vi "Frame Page.vi"(8 "error in (no error)":errorcluster, 11 "Node Ptr":T2 format="%.0x") -> (0 "error out":errorcluster)   [LabVIEW 2019, in "Protection and Counter Addon System Explorer.lvlib"]
uses:
  Protection and Counter Addon System Explorer.lvlib
  <vilib>/NI VeriStand/Custom Device API/Custom Device Item Ref.ctl
  NationalInstruments.VeriStand.SystemStorageUI
  Types/Event Trigger Type.ctl
  <vilib>/NI VeriStand/UI Controls/Single Node Browser/Net Event Data.ctl
  <vilib>/NI VeriStand/UI Controls/Single Node Browser/Net Event.ctl
  Addon Shared/SubVIs/GUID Lookup.vi
  <vilib>/NI VeriStand/Custom Device API/Custom Device API.lvlib
  <vilib>/NI VeriStand/UI Controls/Single Node Browser/NI_VS UI Single Node Browser.lvlib
  Addon Shared/Protection and Counter Addon Shared.lvlib
panel:
  in  "Transmit Trigger":T1
  in  "Trigger":refnum<k24>(container)
  in  "Trigger Settings":cluster{"Section Name":string}={"Section Name"="Transmission Trigger"}
  in  "Trigger":refnum<k24>(container)
  in  "Disable Transmission":bool
  in  "Disable Settings":cluster{"Section Name":string}={"Section Name"="Disable Transmission"}
  in  "Description":string
  out "Frame ID":u32 format="%.0x"
  in  "Custom Device Settings":cluster{"Section Name":string}={"Section Name"="Custom Device Item Settings"}
  out "Name":string
  in  "SHDocVw.IWebBrowser2":refnum<k7>(container)
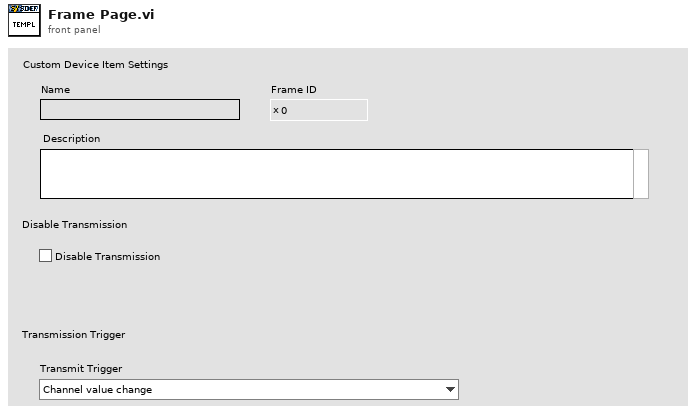
[diagram p1: front panel]
types:
  T1 = typedef "Protection and Counter Addon System Explorer.lvlib/Event Trigger Type.ctl" = enum16{"Channel value change", "Trigger channel (not zero)", "Channel value change or trigger channel (not zero)", "Trigger channel (any value change)", "Channel value change or trigger channel (any value change)"}
  T2 = typedef "Custom Device API.lvlib/Custom Device Item Ref.ctl" = u64
  T3 = cluster{"Trigger":refnum<user-event>, "Transmission":refnum<user-event>}
  T4 = typedef "Protection and Counter Addon System Explorer.lvlib/Frame Settings.ctl" = cluster{"ID":u32, "Disable Transmission":bool, "Disable Transmission Ref":T2, "Transmit Trigger":T1, "Transmit Trigger Ref":T2}
  T5 = typedef "Custom Device API.lvlib/Custom Device Item Info.ctl" = cluster{"Name":string, "Is Channel":bool, "GUID":string, "Is Waveform":bool}
  T6 = typedef "NI_VS UI Single Node Browser.lvlib/Single Node Browser Ref.ctl" = refnum<k24>
  T7 = typedef "NI_VS UI Single Node Browser.lvlib/Callback Type.ctl" = cluster{"Net Callbacks":refnum<k27>[], "Event":refnum<user-event>}
  T8 = typedef "Custom Device API.lvlib/Custom Device Commands.ctl" = enum16{"Default", "Item renamed", "Shutdown", "Dynamic button pressed"}
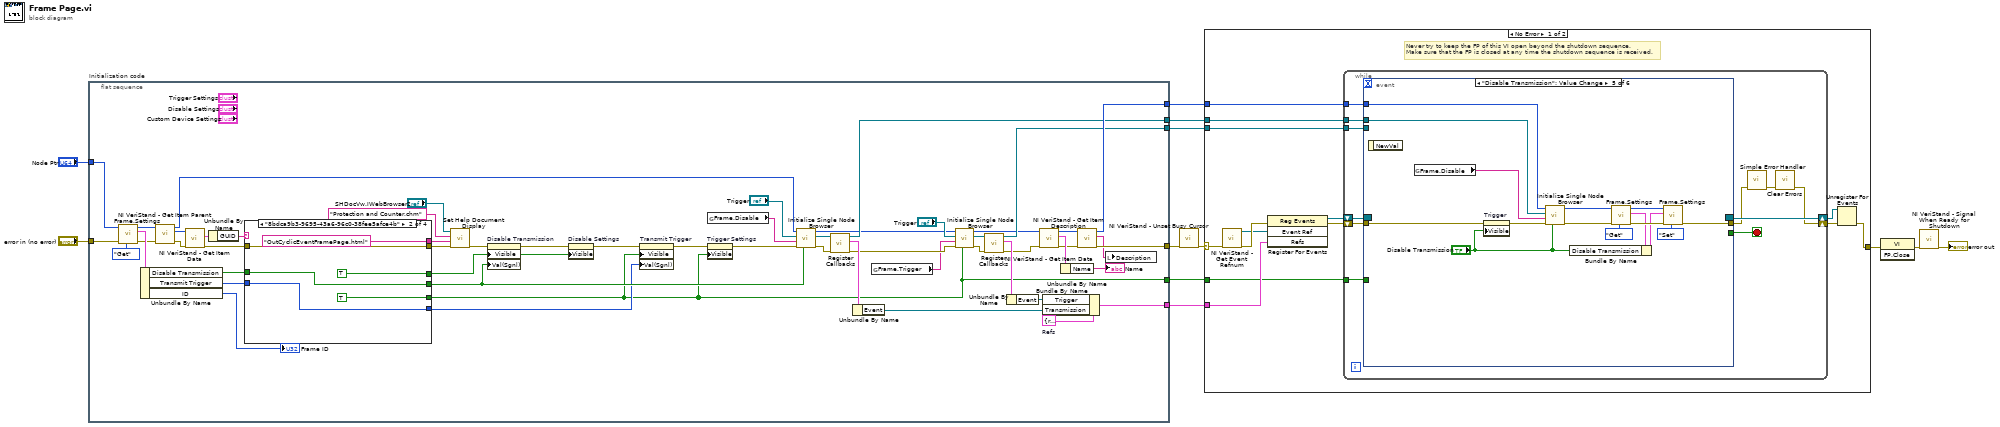
[diagram p0: block diagram]
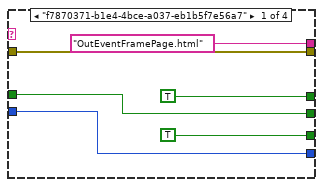
[diagram p2: hidden frame]
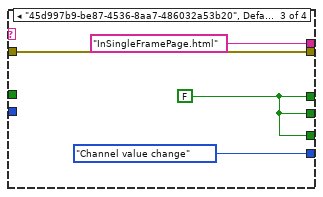
[diagram p3: hidden frame]
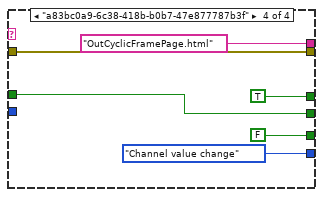
[diagram p4: hidden frame]
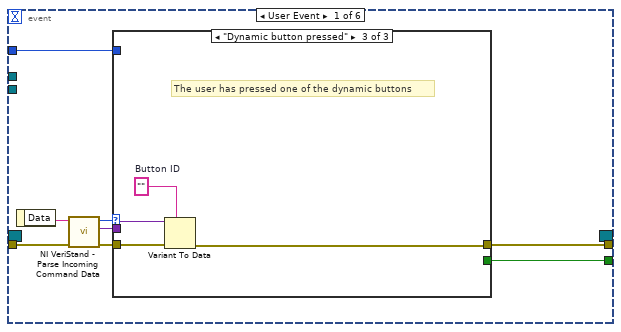
[diagram p5: hidden frame]
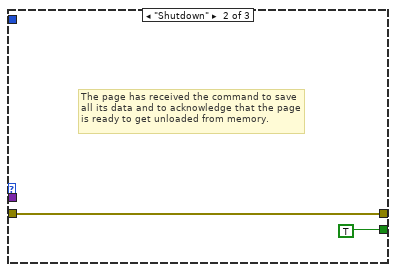
[diagram p7: hidden frame]
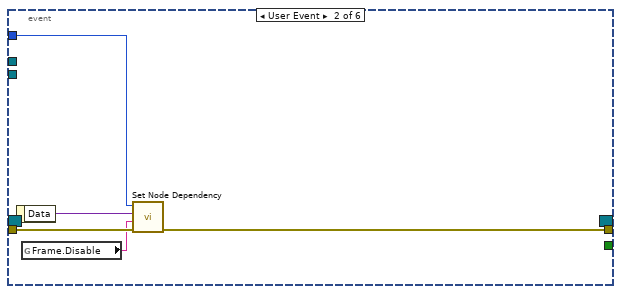
[diagram p8: hidden frame]
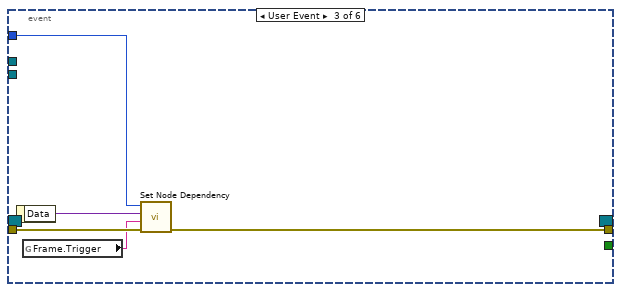
[diagram p9: hidden frame]
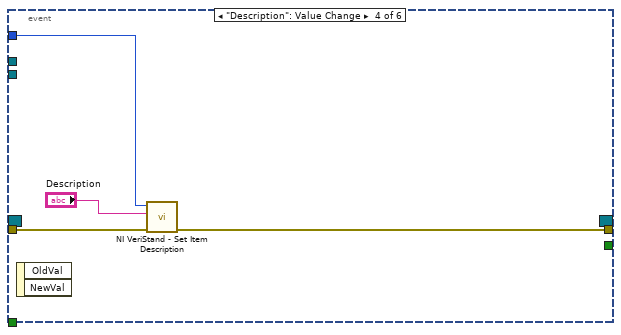
[diagram p10: hidden frame]
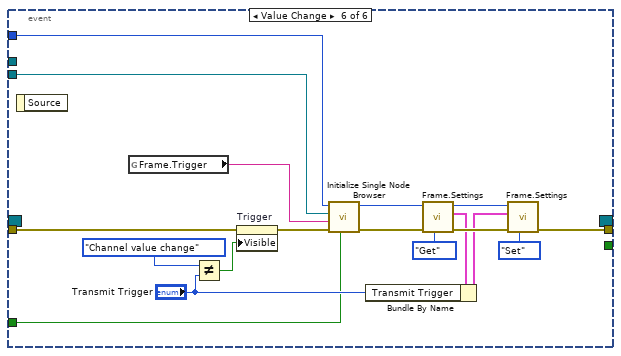
[diagram p11: hidden frame]
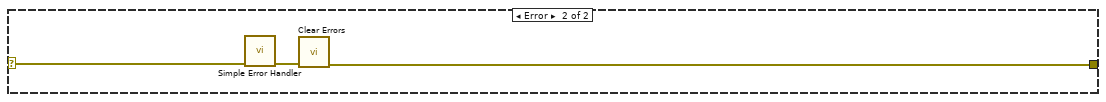
[diagram p12: hidden frame]
diagram:
  n1 = flat-sequence "Initialization code" {
    tunnel: "error in (no error)" -> [w22]
    tunnel: "Node Ptr" -> [w20]
    tunnel: [w61] -> w7
    tunnel: [w59] -> w5
    tunnel: [w43] -> w4
    tunnel: [w45] -> w3
    tunnel: [w35] -> w2
    tunnel: [w15] -> w1
    frame #0 {
      w38 = T3 {"Trigger"=refnum, "Transmission"=refnum}  # Refs
      n2 = call "Frame.Settings.vi"("Action"=enum8{"Get", "Set"}."Get", "error in (no error)"=w22, "Item Ref in"=w20) -> ("error out"=w21:errorcluster, "Frame.Settings"=w26:T4, "Item Ref out"=w19:T2)  [unwired: 6 in]
      n3 = Unbundle By Name(w26) -> ("Disable Transmission"=w18:bool, "Transmit Trigger"=w17:T1, "ID"=→"Frame ID":u32)
      n4 = call <vilib>:"NI VeriStand - Get Item Parent.vi"("error in (no error)"=w21, "Item Ref in"=w19) -> ("error out"=w57:errorcluster, "Parent Ref"=w56:T2, "Item Ref out"=w49:T2)  [unwired: 6 in, 1 out]
      n5 = call <vilib>:"NI VeriStand - Get Item Data.vi"("error in (no error)"=w57, "Item Ref in"=w56) -> ("error out"=w53:errorcluster, "Item Info"=w55:T5)  [unwired: 8 out]
      n6 = Unbundle By Name(w55) -> ("GUID"=w54:string)
      n7 = case shown="\"8bdca9b3-9695-43a6-96c0-38fee5afce4b\"" w54 {
        tunnel: ["OutEventFramePage.html" ("HTML File") "OutCyclicEventFramePage.html" ("HTML File") "InSingleFramePage.html" ("HTML File") "OutCyclicFramePage.html" ("HTML File")] -> w66
        tunnel: w53 -> [w72 w78 w82 w88]
        tunnel: [w72 w78 w82 w88] -> w28
        tunnel: [TRUE TRUE w81 TRUE] -> w46
        tunnel: [w68 w74 w81 w85] -> w30
        tunnel: [TRUE TRUE w81 FALSE] -> w15
        tunnel: [w69 w75 Event_Trigger_Type."Channel value change" ("y") Event_Trigger_Type."Channel value change" ("y")] -> w29
        tunnel: w18 -> [w68 w74 _ w85]
        tunnel: w17 -> [w69 w75 _ _]
        frame "f7870371-b1e4-4bce-a037-eb1b5f7e56a7" {
        }
        frame "8bdca9b3-9695-43a6-96c0-38fee5afce4b" {
        }
        frame "45d997b9-be87-4536-8aa7-486032a53b20", Default {
          w81 = FALSE
        }
        frame "a83bc0a9-6c38-418b-b0b7-47e877787b3f" {
        }
      }
      n8 = call "Set Help Document Display.vi"("error in (no error)"=w28, "HTML File"=w66, "Main CHM File"="Protection and Counter.chm", "SHDocVw.IWebBrowser2"="SHDocVw.IWebBrowser2") -> ("error out"=w27:errorcluster)  [unwired: 7 in]
      n9 = property on="Disable Transmission" class="Bool (strict)"(error in=w27, "Visible"=w46, "Val(Sgnl)"=w30) -> (error out=w52:errorcluster)  [unwired: 1 in, 1 out]
      n10 = property on="Disable Settings" class="Clust (strict)"(error in=w52, "Visible"=w46) -> (error out=w32:errorcluster)  [unwired: 1 in, 1 out]
      n11 = property on="Transmit Trigger" class="Enum (strict)"(error in=w32, "Visible"=w15, "Val(Sgnl)"=w29) -> (error out=w31:errorcluster)  [unwired: 1 in, 1 out]
      n12 = property on="Trigger Settings" class="Clust (strict)"(error in=w31, "Visible"=w15) -> (error out=w33:errorcluster)  [unwired: 1 in, 1 out]
      n13 = global read "GUID Lookup.vi" "Frame.Disable"() -> (w14:string)
      n14 = call "Initialize Single Node Browser.vi"("Use Channel?"=w30, "error in (no error)"=w33, "NodeName"=w14, "Browser Ref 2"="Trigger", "Item Ref in"=w49) -> ("error out"=w51:errorcluster, "Browser Ref"=w50:T6, "Item Ref out"=w34:T2)  [unwired: 4 in]
      n15 = call <vilib>:"Register Callbacks.vi"("error in (no error)"=w51, "Single Node Browser"=w50) -> ("error out"=w39:errorcluster, "Callbacks"=w48:T7, "Single Node Browser dup"=w45:T6)  [unwired: 7 in]
      n16 = Unbundle By Name(w48) -> ("Event"=w44:refnum<user-event>)
      n17 = global read "GUID Lookup.vi" "Frame.Trigger"() -> (w13:string)
      n18 = call "Initialize Single Node Browser.vi"("Use Channel?"=w15, "error in (no error)"=w39, "NodeName"=w13, "Browser Ref 2"="Trigger", "Item Ref in"=w34) -> ("error out"=w40:errorcluster, "Browser Ref"=w41:T6, "Item Ref out"=w23:T2)  [unwired: 4 in]
      n19 = call <vilib>:"Register Callbacks.vi"("error in (no error)"=w40, "Single Node Browser"=w41) -> ("error out"=w24:errorcluster, "Callbacks"=w42:T7, "Single Node Browser dup"=w35:T6)  [unwired: 7 in]
      n20 = Unbundle By Name(w42) -> ("Event"=w37:refnum<user-event>)
      n21 = call <vilib>:"NI VeriStand - Get Item Data.vi"("error in (no error)"=w24, "Item Ref in"=w23) -> ("error out"=w62:errorcluster, "Item Info"=w64:T5, "Item Ref out"=w60:T2)  [unwired: 7 out]
      n22 = Bundle By Name(cluster=w38, "Trigger"=w37, "Transmission"=w44) -> (w43:T3)
      n23 = Unbundle By Name(w64) -> ("Name"=→"Name":string)
      n24 = call <vilib>:"NI VeriStand - Get Item Description.vi"("error in (no error)"=w62, "Item Ref in"=w60) -> ("error out"=w61:errorcluster, "Description"=w58:string, "Item Ref out"=w59:T2)  [unwired: 7 out]
      n25 = local write "Description"(w58) -> ()
    }
  }
  n26 = call <vilib>:"NI VeriStand - Unset Busy Cursor.vi"("error in (no error)"=w7) -> ("error out"=w9:errorcluster)  [unwired: 10 out]
  n27 = case shown="No Error" w9 {
    selector: w9 -> [w94 w178]
    tunnel: [w99 w176] -> w12
    tunnel: w5 -> [w95 _]
    tunnel: w4 -> [w93 _]
    tunnel: w3 -> [w92 _]
    tunnel: w2 -> [w91 _]
    tunnel: w1 -> [w90 _]
    frame No Error {
      # "Never try to keep the FP of this VI open beyond the shutdown sequence.\nMake sure that the FP is closed at any time the shutdown sequence is received."
      n28 = call <vilib>:"NI VeriStand - Get Event Refnum.vi"("error in (no error)"=w94) -> ("error out"=w102:errorcluster, "Event Ref"=w98:refnum<user-event>)  [unwired: 9 out]
      n29 = register-events(error in=w102, w98, w93) -> (reference out=w96:refnum<event-registration>, error out=w97:errorcluster)  [unwired: 1 in]
      n30 = while {
        tunnel: w95 -> [w109]
        shift-right: [w106] -> w100
        shift-left: w97 -> [w112]
        shift-right: [w113] -> w101
        shift-left: w96 -> [w111]
        tunnel: w92 -> [w105]
        tunnel: w91 -> [w104]
        tunnel: w90 -> [w103]
        stop <- w110 stop-if-true
        n31 = event shown="[4] \"Disable Transmission\": Value Change" {
          selector: w111 -> [_ _ _ _ _ _]
          dyn-events: [_ _ _ _ _ _] -> w113
          timeout: _ -> [_ _ _ _ _ _]
          tunnel: w112 -> [w121 w131 w136 w142 w157 w175]
          tunnel: [w117 _ _ _ _ _] -> w110
          tunnel: [w116 w130 w135 w141 w148 w162] -> w108
          tunnel: w109 -> [w115 w132 w137 w140 w155 w174]
          tunnel: w105 -> [_ _ _ _ w156 _]
          tunnel: w104 -> [_ _ _ _ _ w170]
          tunnel: w103 -> [_ _ _ _ _ w160]
          event User Event {
            n32 = event-data() -> ("Data"=w120:string)  [unwired: 1 out]
            n33 = call <vilib>:"NI VeriStand - Parse Incoming Command Data.vi"("error in (no error)"=w121, "Incoming data"=w120) -> ("error out"=w119:errorcluster, "Outgoing data"=w114:variant, "Action"=w118:T8)  [unwired: 7 out]
            n34 = case shown="\"Dynamic button pressed\"" w118 {
              tunnel: w119 -> [w122 w123 w128]
              tunnel: [_ TRUE _] -> w117
              tunnel: [w122 w123 w125] -> w116
              tunnel: w115 -> [_ _ _]
              tunnel: w114 -> [_ _ w127]
              frame "Default", Default {
              }
              frame "Shutdown" {
                # "The page has received the command to save all its data and to acknowledge that the page is ready to get unloaded from memory."
              }
              frame "Dynamic button pressed" {
                w126 = ""  # Button ID
                # "The user has pressed one of the dynamic buttons"
                n35 = Variant To Data(error in=w128, type=w126, Variant=w127) -> (error out=w125:errorcluster)  [unwired: 1 out]
              }
            }
          }
          event User Event {
            n36 = event-data() -> ("Data"=w133:variant)  [unwired: 1 out]
            n37 = global read "GUID Lookup.vi" "Frame.Disable"() -> (w129:string)
            n38 = call "Set Node Dependency.vi"("error in (no error)"=w131, "NodeName"=w129, "Data"=w133, "Item Ref in"=w132) -> ("error out"=w130:errorcluster)  [unwired: 6 in, 1 out]
          }
          event User Event {
            n39 = event-data() -> ("Data"=w138:variant)  [unwired: 1 out]
            n40 = global read "GUID Lookup.vi" "Frame.Trigger"() -> (w134:string)
            n41 = call "Set Node Dependency.vi"("error in (no error)"=w136, "NodeName"=w134, "Data"=w138, "Item Ref in"=w137) -> ("error out"=w135:errorcluster)  [unwired: 6 in, 1 out]
          }
          event "Description": Value Change {
            n42 = event-data() -> ()  [unwired: 3 out]
            n43 = call <vilib>:"NI VeriStand - Set Item Description.vi"("error in (no error)"=w142, "Description"="Description", "Item Ref in"=w140) -> ("error out"=w141:errorcluster)  [unwired: 8 out]
          }
          event "Disable Transmission": Value Change {
            n44 = event-data() -> ()  [unwired: 2 out]
            n45 = global read "GUID Lookup.vi" "Frame.Disable"() -> (w143:string)
            n46 = property on="Trigger" class="AXCont"(error in=w157, "Visible"="Disable Transmission") -> (error out=w154:errorcluster)  [unwired: 1 in, 1 out]
            n47 = call "Initialize Single Node Browser.vi"("Use Channel?"="Disable Transmission", "error in (no error)"=w154, "NodeName"=w143, "Browser Ref 2"=w156, "Item Ref in"=w155) -> ("error out"=w151:errorcluster, "Item Ref out"=w152:T2)  [unwired: 4 in, 1 out]
            n48 = call "Frame.Settings.vi"("Action"=enum8{"Get", "Set"}."Get", "error in (no error)"=w151, "Item Ref in"=w152) -> ("error out"=w149:errorcluster, "Frame.Settings"=w146:T4, "Item Ref out"=w147:T2)  [unwired: 6 in]
            n49 = Bundle By Name(cluster=w146, "Disable Transmission"="Disable Transmission") -> (w144:T4)
            n50 = call "Frame.Settings.vi"("Action"=enum8{"Get", "Set"}."Set", "error in (no error)"=w149, "Frame.Settings"=w144, "Item Ref in"=w147) -> ("error out"=w148:errorcluster)  [unwired: 5 in, 2 out]
          }
          event Value Change {
            n51 = event-data() -> ()  [unwired: 2 out]
            n52 = global read "GUID Lookup.vi" "Frame.Trigger"() -> (w158:string)
            n53 = Not Equal?(x=Event_Trigger_Type."Channel value change" ("y"), y="Transmit Trigger") -> (x != y?=w171:bool)
            n54 = property on="Trigger" class="AXCont"(error in=w175, "Visible"=w171) -> (error out=w173:errorcluster)  [unwired: 1 in, 1 out]
            n55 = call "Initialize Single Node Browser.vi"("Use Channel?"=w160, "error in (no error)"=w173, "NodeName"=w158, "Browser Ref 2"=w170, "Item Ref in"=w174) -> ("error out"=w163:errorcluster, "Item Ref out"=w161:T2)  [unwired: 4 in, 1 out]
            n56 = call "Frame.Settings.vi"("Action"=enum8{"Get", "Set"}."Get", "error in (no error)"=w163, "Item Ref in"=w161) -> ("error out"=w167:errorcluster, "Frame.Settings"=w165:T4, "Item Ref out"=w166:T2)  [unwired: 6 in]
            n57 = Bundle By Name(cluster=w165, "Transmit Trigger"="Transmit Trigger") -> (w159:T4)
            n58 = call "Frame.Settings.vi"("Action"=enum8{"Get", "Set"}."Set", "error in (no error)"=w167, "Frame.Settings"=w159, "Item Ref in"=w166) -> ("error out"=w162:errorcluster)  [unwired: 5 in, 2 out]
          }
        }
        n59 = call <vilib>:"Simple Error Handler.vi"("error in (no error)"=w108) -> ("error out"=w107:errorcluster)  [unwired: 1 in, 7 out]
        n60 = call <vilib>:"Clear Errors.vi"("error in (no error)"=w107) -> ("error out"=w106:errorcluster)  [unwired: 1 in, 5 out]
      }
      n61 = Unregister For Events(event registration refnum=w101, error in=w100) -> (error out=w99:errorcluster)
    }
    frame Error {
      n62 = call <vilib>:"Simple Error Handler.vi"("error in (no error)"=w178) -> ("error out"=w177:errorcluster)  [unwired: 1 in, 7 out]
      n63 = call <vilib>:"Clear Errors.vi"("error in (no error)"=w177) -> ("error out"=w176:errorcluster)  [unwired: 1 in, 5 out]
    }
  }
  n64 = invoke class="VI" method="FP.Close"(error in=w12) -> (error out=w11:errorcluster)  [unwired: 2 in, 2 out]
  n65 = call <vilib>:"NI VeriStand - Signal When Ready for Shutdown.vi"("error in (no error)"=w11) -> ("error out"=→"error out":errorcluster)  [unwired: 10 out]
